vi "RetaInimigoBola.vi"(1 "DistInFrontGoal":dbl=90.0 format="%#_13g", 4 "Y quina":dbl format="%#_13g", 5 "Meio?":bool=TRUE, 6 "Goal width":u32, 7 "Field lenght":u32, 8 "Y bola":dbl format="%#_13g", 9 "X bola":dbl format="%#_13g", 10 "Y inimigo":dbl format="%#_13g", 11 "X inimigo":dbl format="%#_13g") -> (0 "Orientação":dbl format="%#_13g", 2 "Y goleiro":dbl format="%#_13g", 3 "X goleiro":dbl format="%#_13g")   [LabVIEW 2023]
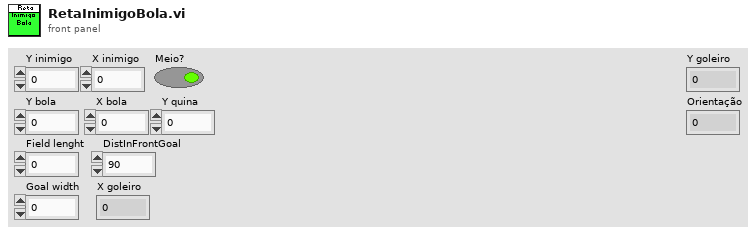
[diagram p1: front panel]
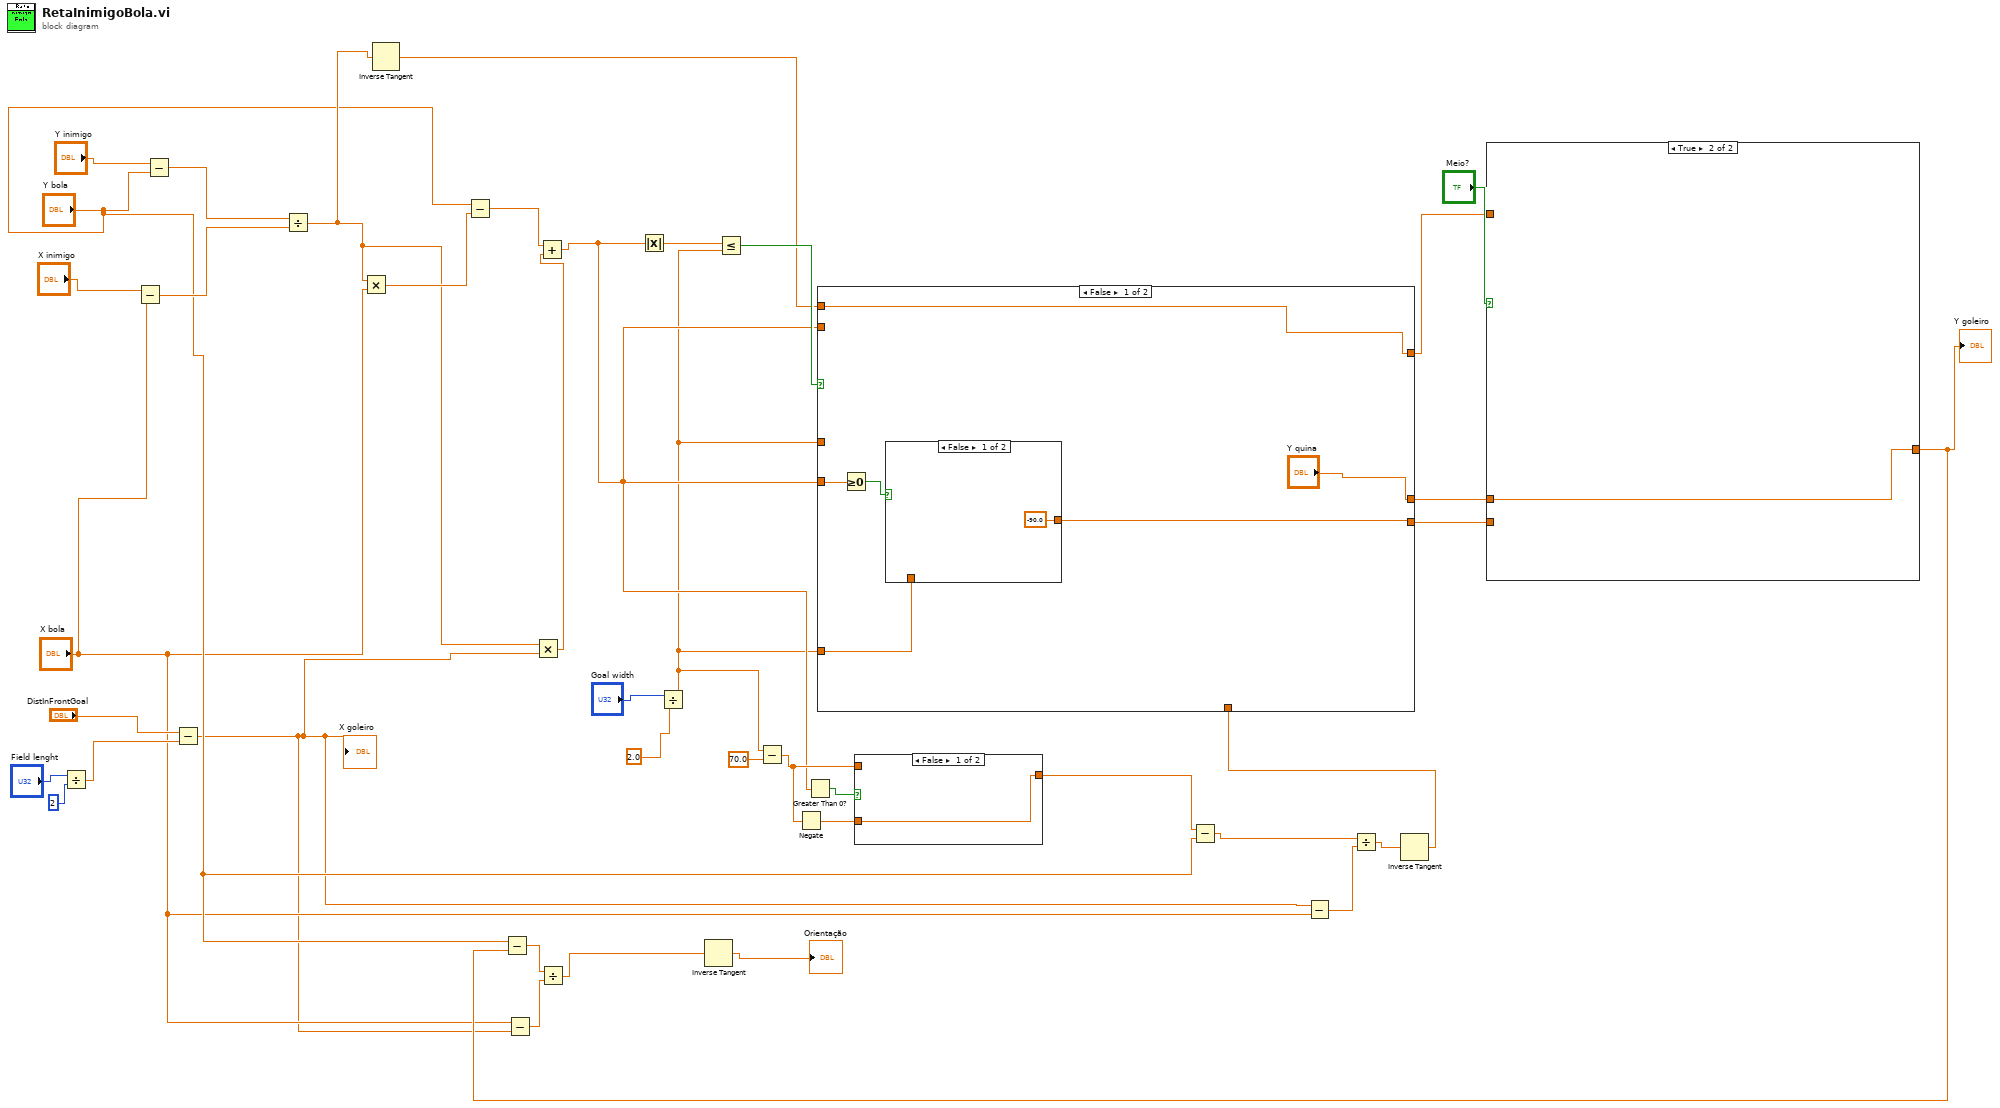
[diagram p0: block diagram]
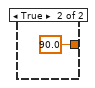
[diagram p4: hidden frame]
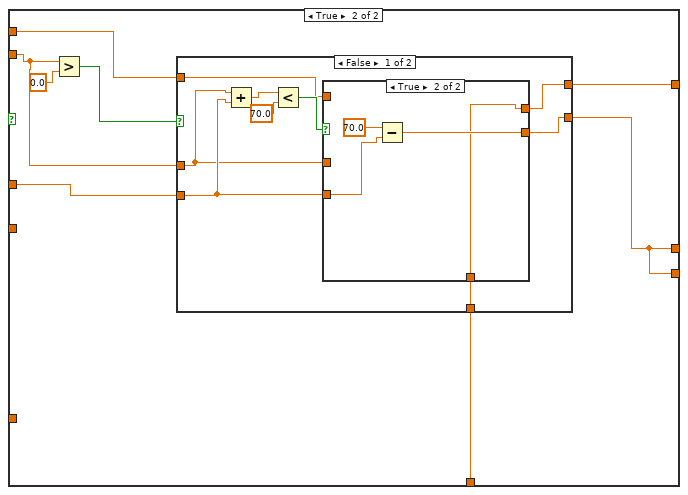
[diagram p5: hidden frame]
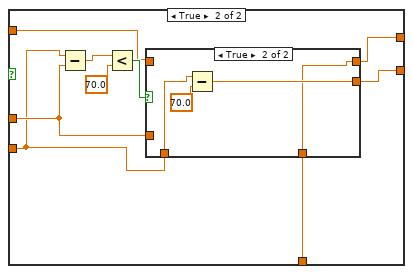
[diagram p7: hidden frame]
diagram:
  n1 = Divide(x="Field lenght", y=2) -> (x/y=w32:dbl)
  n2 = Subtract(x="X inimigo", y="X bola") -> (x-y=w37:dbl)
  n3 = Subtract(x="Y inimigo", y="Y bola") -> (x-y=w38:dbl)
  n4 = Subtract(x="DistInFrontGoal", y=w32) -> (x-y=w1:dbl)
  "X goleiro" <- w1
  n5 = Divide(x=w38, y=w37) -> (x/y=w25:dbl)
  n6 = Multiply(x=w25, y="X bola") -> (x*y=w36:dbl)
  n7 = Inverse Tangent(1:w25) -> (0:w24:dbl)
  n8 = Subtract(x="Y bola", y=w36) -> (x-y=w31:dbl)
  n9 = Subtract(x="X bola", y=w1) -> (x-y=w3:dbl)
  n10 = Multiply(x=w25, y=w1) -> (x*y=w30:dbl)
  n11 = Add(x=w31, y=w30) -> (x+y=w10:dbl)
  n12 = Absolute Value(x=w10) -> (abs(x)=w29:dbl)
  n13 = Divide(x="Goal width", y=2.0) -> (x/y=w9:dbl)
  n14 = Less Or Equal?(x=w29, y=w9) -> (x <= y?=w28:bool)
  n15 = Subtract(x=w9, y=70.0) -> (x-y=w20:dbl)
  n16 = Negate(x=w20) -> (-x=w19:dbl)
  n17 = Greater Than 0?(x=w10) -> (x > 0?=w22:bool)
  n18 = case shown="False" w22 {
    tunnel: w20 -> [_ w42]
    tunnel: [w41 w42] -> w21
    tunnel: w19 -> [w41 _]
    frame False {
    }
    frame True {
    }
  }
  n19 = Subtract(x=w21, y="Y bola") -> (x-y=w18:dbl)
  n20 = Subtract(x=w1, y="X bola") -> (x-y=w17:dbl)
  n21 = Divide(x=w18, y=w17) -> (x/y=w16:dbl)
  n22 = Inverse Tangent(1:w16) -> (0:w15:dbl)
  n23 = case shown="False" w28 {
    tunnel: ["Y quina" w51] -> w12
    tunnel: w10 -> [_ w55]
    tunnel: w9 -> [_ w56]
    tunnel: w24 -> [w48 w54]
    tunnel: [w48 w53] -> w13
    tunnel: w15 -> [_ w52]
    tunnel: [w44 w51] -> w11
    tunnel: w10 -> [w47 _]
    tunnel: w9 -> [w45 _]
    frame False {
      n24 = Greater Or Equal To 0?(x=w47) -> (x >= 0?=w46:bool)
      n25 = case shown="False" w46 {
        tunnel: w45 -> [_ _]
        tunnel: [-90.0 90.0] -> w44
        frame False {
        }
        frame True {
        }
      }
    }
    frame True {
      n26 = Greater?(x=w55, y=0.0) -> (0:w57:bool)
      n27 = case shown="False" w57 {
        tunnel: w56 -> [w64 w77]
        tunnel: w55 -> [w62 w78]
        tunnel: [w63 w79] -> w51
        tunnel: w54 -> [w61 w76]
        tunnel: [w60 w75] -> w53
        tunnel: w52 -> [w59 w74]
        frame False {
          n28 = Add(x=w62, y=w64) -> (x+y=w67:dbl)
          n29 = Less?(x=w67, y=70.0) -> (x < y?=w65:bool)
          n30 = case shown="True" w65 {
            tunnel: w64 -> [_ w72]
            tunnel: [w69 w71] -> w63
            tunnel: w62 -> [w69 _]
            tunnel: w61 -> [w68 _]
            tunnel: [w68 w70] -> w60
            tunnel: w59 -> [_ w70]
            frame False {
            }
            frame True {
              n31 = Subtract(x=70.0, y=w72) -> (x-y=w71:dbl)
            }
          }
        }
        frame True {
          n32 = Subtract(x=w77, y=w78) -> (x-y=w82:dbl)
          n33 = Less?(x=w82, y=70.0) -> (x < y?=w80:bool)
          n34 = case shown="True" w80 {
            tunnel: [w84 w87] -> w79
            tunnel: w78 -> [w84 _]
            tunnel: w77 -> [_ w86]
            tunnel: w76 -> [w83 _]
            tunnel: [w83 w85] -> w75
            tunnel: w74 -> [_ w85]
            frame False {
            }
            frame True {
              n35 = Subtract(x=w86, y=70.0) -> (x-y=w87:dbl)
            }
          }
        }
      }
    }
  }
  n36 = case shown="True" "Meio?" {
    tunnel: w13 -> [_ _]
    tunnel: [w89 w90] -> w7
    tunnel: w12 -> [_ w90]
    tunnel: w11 -> [w89 _]
    frame False {
    }
    frame True {
    }
  }
  "Y goleiro" <- w7
  n37 = Subtract(x="Y bola", y=w7) -> (x-y=w4:dbl)
  n38 = Divide(x=w4, y=w3) -> (x/y=w2:dbl)
  n39 = Inverse Tangent(1:w2) -> (0:→"Orientação":dbl)
